vi "SftpInitialize.vi"(0 "error in":errorcluster, 9 "Username":string, 11 "Password":string) -> (4 "error out":errorcluster, 15 "SFTP Connect Parameters":refnum<k24>)   [LabVIEW 2015, in "UnderAutomation.UniversalRobots.lvlib"]
uses:
  UnderAutomation.UniversalRobots.lvlib
  C:/Users/fg/Documents/UniversalRobots.vi/LabVIEW_2024/UnderAutomation.UniversalRobots/lib/UnderAutomation.UniversalRobots.dll
  LabVIEW_2024/UnderAutomation.UniversalRobots/lib/UnderAutomation.UniversalRobots.dll
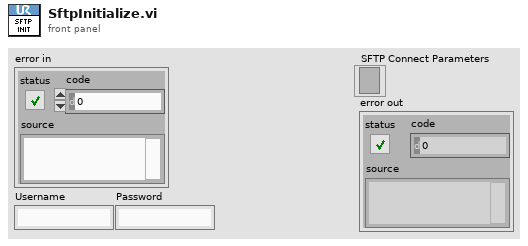
[diagram p1: front panel]
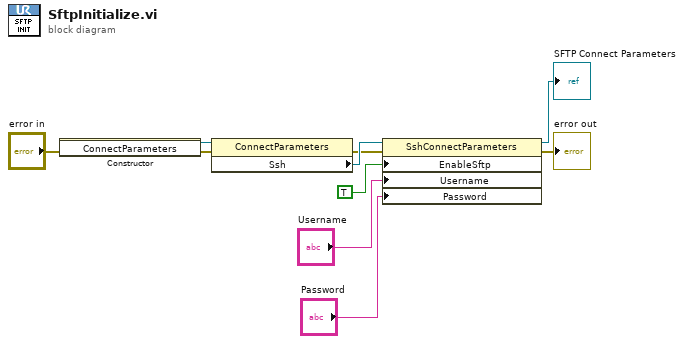
[diagram p0: block diagram]
diagram:
  n1 = constructor class="ConnectParameters"(error in="error in") -> (reference out=w10:refnum<k24>, error out=w8:errorcluster)  [unwired: 2 in, 1 out]
  n2 = property class="ConnectParameters"(reference=w10, error in=w8) -> (error out=w6:errorcluster, "Ssh"=w7:refnum<k24>)  [unwired: 1 out]
  n3 = property class="SshConnectParameters"(reference=w7, error in=w6, "EnableSftp"=TRUE, "Username"="Username", "Password"="Password") -> (reference out=→"SFTP Connect Parameters":refnum<k24>, error out=→"error out":errorcluster)
